vi "send command to printer( Serial ).vi"(8 "error in (no error)":errorcluster, 10 "command to be sent":string, 11 "Domino Laser module Class in":refnum<class "Domino Laser module Class.lvclass">) -> (0 "error out":errorcluster, 1 "Command Excuted succeddfully?":bool, 2 "Recived message":string, 3 "Domino Laser module Class out":refnum<class "Domino Laser module Class.lvclass">)   [LabVIEW 2024, in "Domino LM.lvlib"]
uses:
  Domino LM.lvlib
  CTRLS/Domino Laser module Class.lvclass
  CTRLS/Domino Laser module Class.lvclass/Domino Laser module Class.ctl
panel:
  out "Recived":string[](array[string])
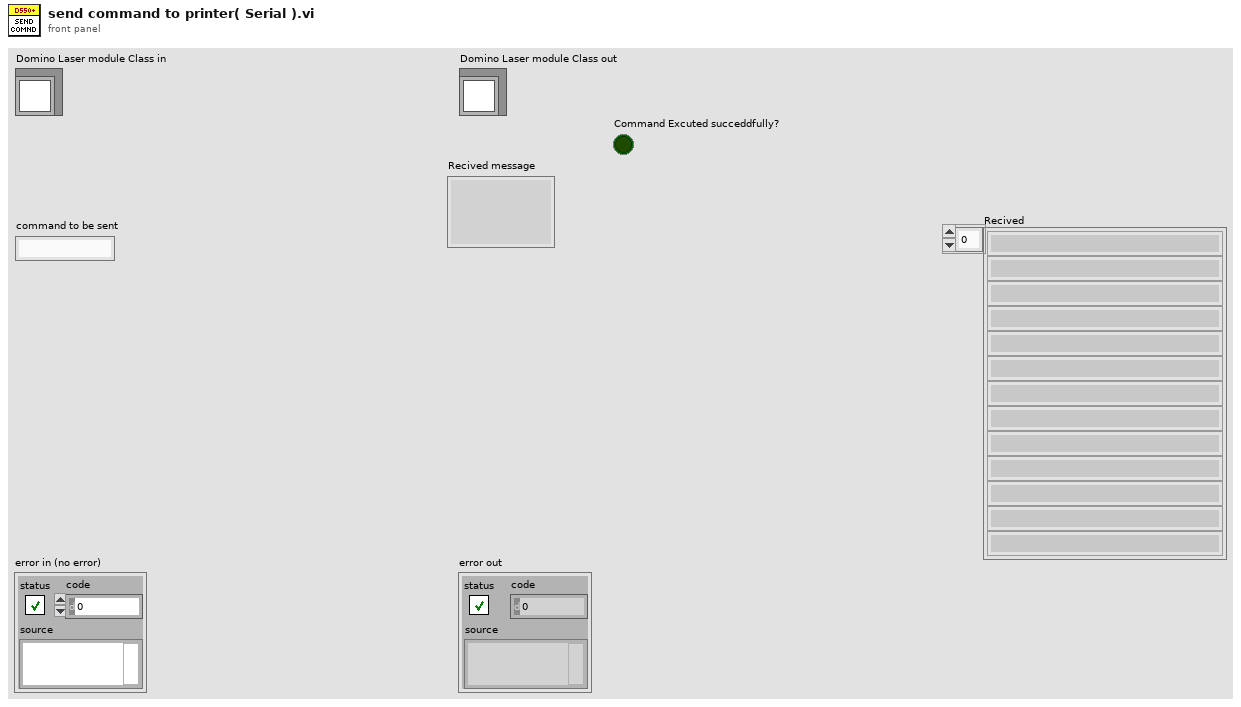
[diagram p1: front panel]
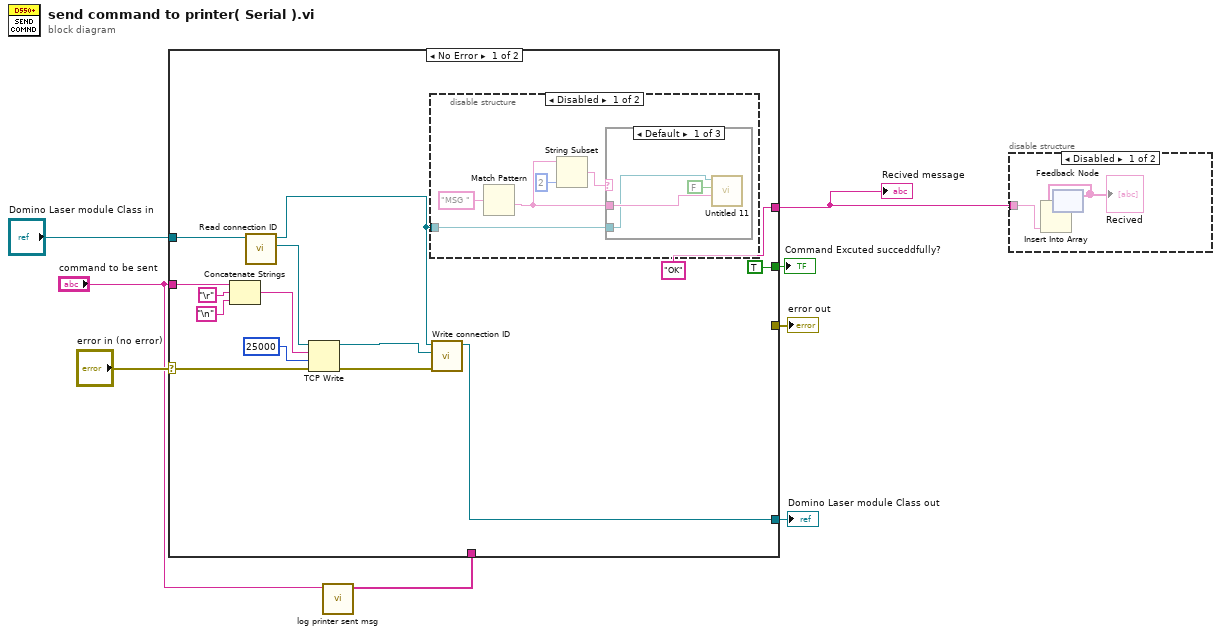
[diagram p0: block diagram]
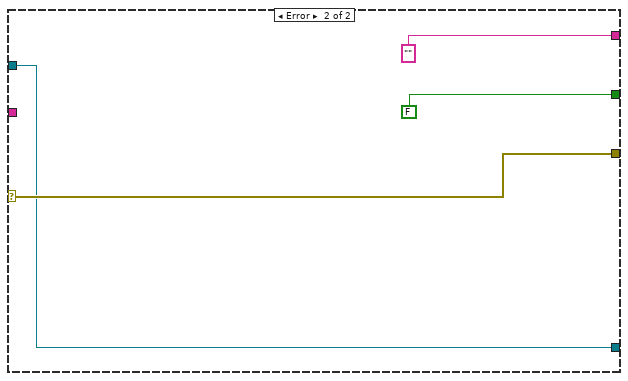
[diagram p6: hidden frame]
diagram:
  n1 = call "log printer sent msg.vi"("new element/subarray"="command to be sent") -> ("sent 2"=w1:string[])  [unwired: 9 in, 1 out]
  n2 = case shown="No Error" "error in (no error)" {
    selector: "error in (no error)" -> [w16 w34]
    tunnel: [_ w34] -> w7
    tunnel: [w11 w33] -> w5
    tunnel: "Domino Laser module Class in" -> [w15 w33]
    tunnel: ["OK" ("data out") "" ("data out")] -> w3
    tunnel: "command to be sent" -> [w17 _]
    tunnel: [TRUE ("Command Excuted succeddfully?") FALSE ("Command Excuted succeddfully?")] -> w4
    tunnel: w1 -> [_ _]
    frame No Error {
      n3 = Concatenate Strings(w17, "\r", "\n") -> (w19:string)
      n4 = call "Read connection ID.vi"("Domino Laser module Class in"=w15) -> ("connection ID"=w20:refnum<k5>, "Domino Laser module Class out"=w14:refnum<class "Domino Laser module Class.lvclass">)  [unwired: 8 in, 1 out]
      n5 = TCP Write(connection ID=w20, data in=w19, error in (no error)=w16, 9:25000 ("timeout ms (25000)")) -> (connection ID out=w13:refnum<k5>, error out=w12:errorcluster)  [unwired: 1 out]
      n6 = disable-structure shown="Disabled" {
        disable-tunnel: w14 -> [w26 _]
        frame Disabled {
          n7 = Match Pattern(regular expression="MSG ") -> (after substring=w25:string)  [unwired: 2 in, 3 out]
          n8 = String Subset(string=w25, length (rest)=2 ("length (rest)")) -> (substring=w23:string)  [unwired: 1 in]
          n9 = case shown="Default" w23 {
            tunnel: w25 -> [w30 _ _]
            tunnel: w26 -> [w29 _ _]
            frame Default {
              n10 = call "Untitled 11.vi"("MSG"=w30, "MSG Status"=FALSE, "Domino Laser module Class in"=w29) -> ()  [unwired: 7 in, 2 out]
            }
            frame "25" {
            }
            frame "" {
            }
          }
        }
        frame Enabled {
        }
      }
      n11 = call "Write connection ID.vi"("error in (no error)"=w12, "connection ID"=w13, "Domino Laser module Class in"=w14) -> ("Domino Laser module Class out"=w11:refnum<class "Domino Laser module Class.lvclass">)  [unwired: 7 in, 1 out]
    }
    frame Error {
    }
  }
  "error out" <- w7
  "Domino Laser module Class out" <- w5
  "Recived message" <- w3
  "Command Excuted succeddfully?" <- w4
  n12 = disable-structure shown="Disabled" {
    disable-tunnel: w3 -> [w37 _]
    frame Disabled {
      n13 = feedback #1() -> (w35:string[])  [unwired: 1 in]
      "Recived" <- w35
      n14 = Insert Into Array(array=w35, new element=w37) -> (w36:string[])  [unwired: 1 in]
      n15 = feedback-in #1(w36) -> ()
    }
    frame Enabled {
    }
  }
